vi "Spectrograph_acceptCommand_moveLinearStage.vi"(8 "error in (no error)":errorcluster, 11 "command_moveLinearStage_Ctl":T1) -> (0 "error out":errorcluster, 2 "function return":i32, 3 "command_moveLinearStage_Ctl out":T1)   [LabVIEW 2016, in "SALLV_Spectrograph.lvlib"]
doc: "int Spectrograph_shm_acceptCommand_moveLinearStageLV(Spectrograph_command_moveLinearStageLV *command_moveLinearStage_Ctl );"
uses:
  SALLV_Spectrograph.lvlib
  DataTypes/command_moveLinearStage.ctl
  SALLV_Spectrograph.so
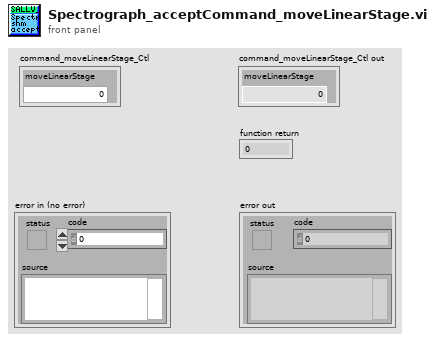
[diagram p1: front panel]
types:
  T1 = typedef "SALLV_Spectrograph.lvlib/command_moveLinearStage.ctl" = cluster{"moveLinearStage":dbl}
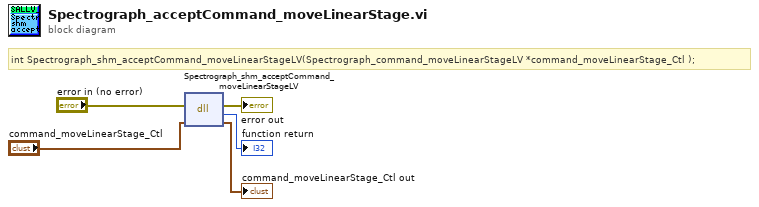
[diagram p0: block diagram]
diagram:
  # "int Spectrograph_shm_acceptCommand_moveLinearStageLV(Spectrograph_command_moveLinearStageLV *command_moveLinearStage_Ctl );"
  n1 = dll-call lib="home/harini/TCS/SALLV_Spectrograph/SALLV_Spectrograph.*" fn="Spectrograph_shm_acceptCommand_moveLinearStageLV"(error in="error in (no error)", "command_moveLinearStage_Ctl"="command_moveLinearStage_Ctl") -> (error out=→"error out":errorcluster, →"function return":i32, "command_moveLinearStage_Ctl"=→"command_moveLinearStage_Ctl out":T1)  [unwired: 2 in, 1 out]
